vi "FG Set State.vi"(7 "Force to continuous mode?":bool, 8 "error in (no error)":errorcluster, 9 "voltage (Vpp)":dbl[unit], 10 "Channel (0: Channel 1)":T1 items=["Channel 1", "Channel 2"], 11 "VISA resource name":refnum<visa-resource-name>) -> (0 "error out":errorcluster, 3 "VISA resource name out":refnum<visa-resource-name>)   [LabVIEW 2009]
uses:
  Tektronix AFG 3000 Series/controls.llb/Channel.ctl
  Tektronix AFG 3000 Series/controls.llb/Frequency Mode.ctl
  Tektronix AFG 3000 Series/controls.llb/Waveform Shape.ctl
  Tektronix AFG 3000 Series/controls.llb/Volt Unit.ctl
  Tektronix AFG 3000 Series/controls.llb/Voltage.ctl
  Tektronix AFG 3000 Series/Tektronix AFG 3000 Series.lvlib
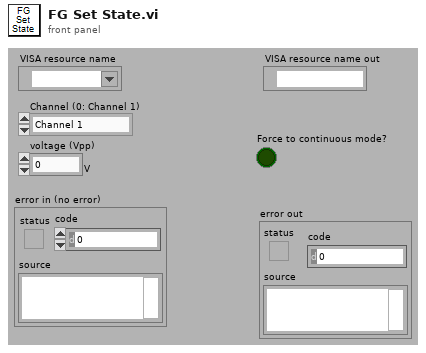
[diagram p1: front panel]
types:
  T1 = typedef "Channel.ctl" = u16
  T2 = typedef "Voltage.ctl" = enum16{"amplitude", "offset", "high", "low", "high limit", "low limit"}
  T3 = typedef "Volt Unit.ctl" = enum16{"VPP", "VRMS", "DBM"}
  T4 = typedef "Waveform Shape.ctl" = u16
  T5 = typedef "Frequency Mode.ctl" = enum16{"CW", "Sweep"}
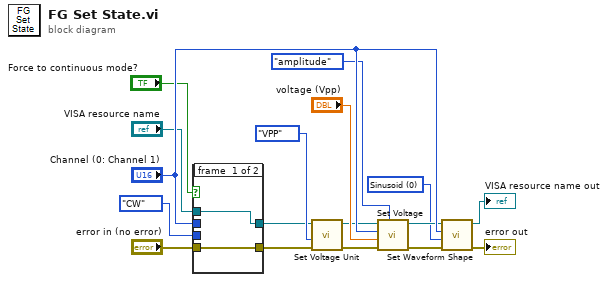
[diagram p0: block diagram]
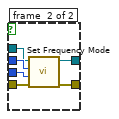
[diagram p2: hidden frame]
diagram:
  w12 = T4 0 items=["Sinusoid", "Square", "Pulse", "Ramp", "PRNoise", "DC", "SINC", "Gaussian", "Lorentz", "ERise", "EDecay", "Haversine", "User 1", "User 2", "User 3", "User 4", "EMemory", "EFile"] ("Waveform Shape")
  n1 = case shown="True" "Force to continuous mode?" {
    tunnel: "Channel (0: Channel 1)" -> [_ w25]
    tunnel: "VISA resource name" -> [w19 w24]
    tunnel: Frequency_Mode."CW" ("Mode (0: CW)") -> [_ w23]
    tunnel: "error in (no error)" -> [w18 w22]
    tunnel: [w19 w21] -> w7
    tunnel: [w18 w20] -> w5
    frame #0 {
    }
    frame #1 {
      n2 = call "Set Frequency Mode.vi"("error in (no error)"=w22, "Mode (0: CW)"=w23, "Channel (0: Channel 1)"=w25, "VISA resource name"=w24) -> ("error out"=w20:errorcluster, "VISA resource name out"=w21:refnum<visa-resource-name>)  [unwired: 6 out]
    }
  }
  n3 = call "Set Voltage Unit.vi"("error in (no error)"=w5, "Volt Unit (VPP)"=Volt_Unit."VPP", "VISA resource name"=w7) -> ("error out"=w4:errorcluster, "VISA resource name out"=w6:refnum<visa-resource-name>)  [unwired: 1 in, 6 out]
  n4 = call "Set Voltage.vi"("Voltage Param (amplitude)"=Voltage."amplitude", "error in (no error)"=w4, "voltage"="voltage (Vpp)", "Channel (0: Channel 1)"="Channel (0: Channel 1)", "VISA resource name"=w6) -> ("error out"=w15:errorcluster, "VISA resource name out"=w16:refnum<visa-resource-name>)  [unwired: 5 out]
  n5 = call "Set Waveform Shape.vi"("error in (no error)"=w15, "Waveform Shape"=w12, "Channel (0: Channel 1)"="Channel (0: Channel 1)", "VISA resource name"=w16) -> ("error out"=→"error out":errorcluster, "VISA resource name out"=→"VISA resource name out":refnum<visa-resource-name>)  [unwired: 6 out]
